vi "niFpgaFFTButterfly.vi"(0 "X in":T1, 2 "stage":u8, 5 "Y in":T1, 7 "TwiddleFactor":T1, 9 "flag":fxp<+,2,2>) -> (4 "X out":T1, 10 "Y out":T1)   [LabVIEW 2017]
uses:
  <vilib>/rvi/FXPMathLib/FxpMul/XNode/nifxpmath_Multiplier.xnode
  <vilib>/rvi/FXPMathLib/basic elements/FxpDiscreteDelay/XNode/nifxpmath_DiscreteDelay.xnode
  <vilib>/rvi/FXPMathLib/sim/FxpSim.dll
types:
  T1 = cluster{"Real":fxp<+/-,16,1>, "Imaginary":fxp<+/-,16,1>}
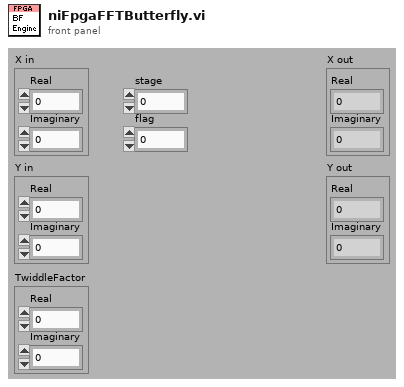
[diagram p1: front panel]
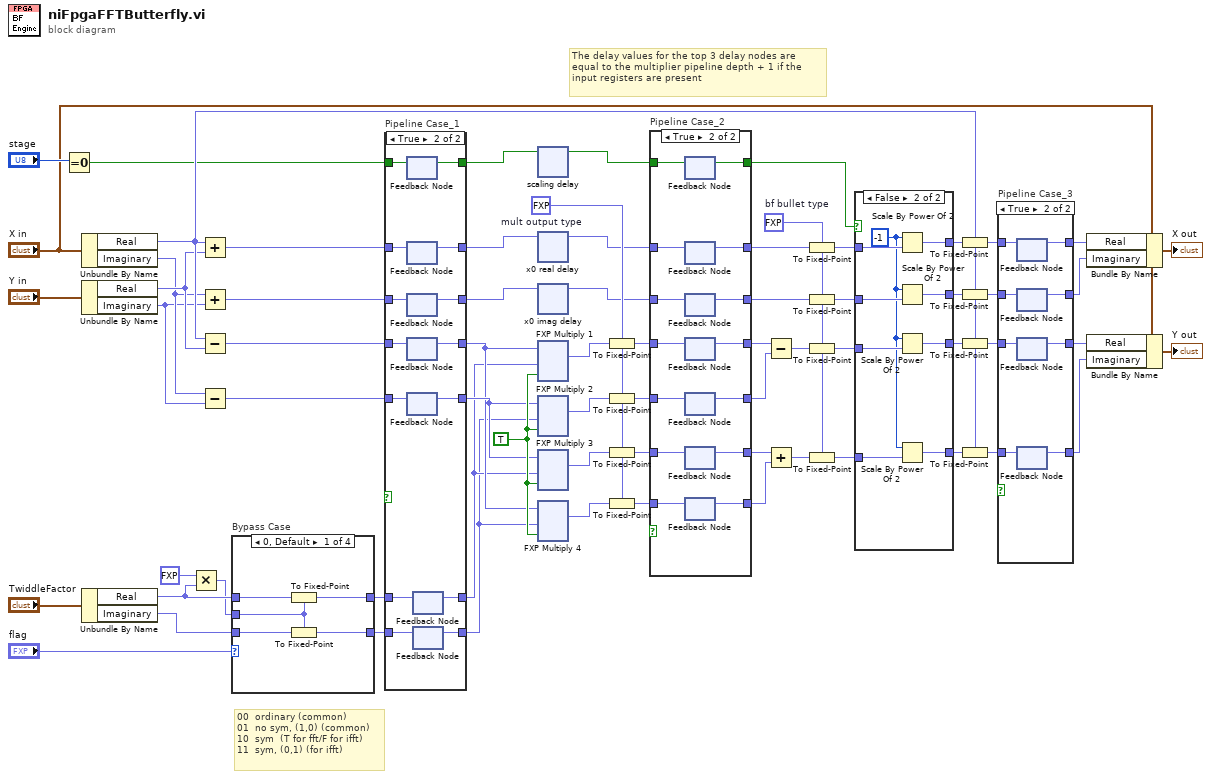
[diagram p0: block diagram]
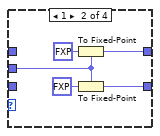
[diagram p5: hidden frame]
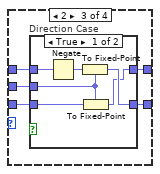
[diagram p6: hidden frame]
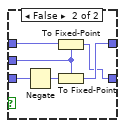
[diagram p7: hidden frame]
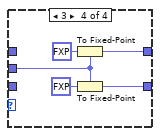
[diagram p8: hidden frame]
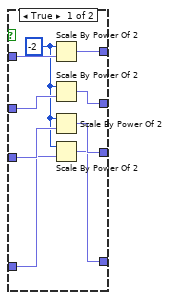
[diagram p9: hidden frame]
diagram:
  w39 = fxp<+/-,18,2> 0.0  # mult output type
  w54 = fxp<+/-,22,4> 0.0  # bf bullet type
  w38 = TRUE ("input valid")
  # "The delay values for the top 3 delay nodes are equal to the multiplier pipeline depth + 1 if the input registers are present"
  # "00  ordinary (common)\n01  no sym, (1,0) (common)\n10  sym  (T for fft/F for ifft)\n11  sym, (0,1) (for ifft)"
  n1 = Equal To 0?(x="stage") -> (x = 0?=w12:bool)
  n2 = Unbundle By Name("X in") -> ("Real"=w48:fxp<+/-,16,1>, "Imaginary"=w46:fxp<+/-,16,1>)
  n3 = Unbundle By Name("Y in") -> ("Real"=w47:fxp<+/-,16,1>, "Imaginary"=w45:fxp<+/-,16,1>)
  n4 = Unbundle By Name("TwiddleFactor") -> ("Real"=w50:fxp<+/-,16,1>, "Imaginary"=w52:fxp<+/-,16,1>)
  n5 = Multiply(x=fxp<+/-,2,2> 0.0, y=w50) -> (x*y=w49:fxp<+/-,17,2>)
  n6 = Add(x=w48, y=w47) -> (x+y=w10:fxp<+/-,17,2>)
  n7 = Add(x=w46, y=w45) -> (x+y=w9:fxp<+/-,17,2>)
  n8 = Subtract(x=w48, y=w47) -> (x-y=w29:fxp<+/-,17,2>)
  n9 = Subtract(x=w46, y=w45) -> (x-y=w30:fxp<+/-,17,2>)
  n10 = case "Bypass Case" shown="0, Default" "flag" {
    tunnel: w50 -> [w73 _ w83 _]
    tunnel: [w72 w77 w79 w99] -> w31
    tunnel: w52 -> [w71 _ w80 _]
    tunnel: [w70 w75 w82 w97] -> w32
    tunnel: w49 -> [w69 w74 w81 w96]
    frame 0, Default {
      n11 = To Fixed-Point(fixed-point type=w69, number=w73) -> (fixed-point=w72:fxp<+/-,17,2>)
      n12 = To Fixed-Point(fixed-point type=w69, number=w71) -> (fixed-point=w70:fxp<+/-,17,2>)
    }
    frame 1 {
      n13 = To Fixed-Point(fixed-point type=w74, number=fxp<+,1,1> 1.0 ("fixed-point type")) -> (fixed-point=w77:fxp<+/-,17,2>)
      n14 = To Fixed-Point(fixed-point type=w74, number=fxp<+,1,1> 0.0 ("fixed-point type")) -> (fixed-point=w75:fxp<+/-,17,2>)
    }
    frame 2 {
      n15 = case "Direction Case" shown="True" {
        selector: _ -> [_ _]
        tunnel: w83 -> [w88 w92]
        tunnel: [w87 w90] -> w82
        tunnel: w81 -> [w86 w94]
        tunnel: w80 -> [w85 w93]
        tunnel: [w84 w91] -> w79
        frame True {
          n16 = Negate(x=w88) -> (-x=w89:fxp<+/-,17,2>)
          n17 = To Fixed-Point(fixed-point type=w86, number=w89) -> (fixed-point=w87:fxp<+/-,17,2>)
          n18 = To Fixed-Point(fixed-point type=w86, number=w85) -> (fixed-point=w84:fxp<+/-,17,2>)
        }
        frame False {
          n19 = Negate(x=w93) -> (-x=w95:fxp<+/-,17,2>)
          n20 = To Fixed-Point(fixed-point type=w94, number=w92) -> (fixed-point=w90:fxp<+/-,17,2>)
          n21 = To Fixed-Point(fixed-point type=w94, number=w95) -> (fixed-point=w91:fxp<+/-,17,2>)
        }
      }
    }
    frame 3 {
      n22 = To Fixed-Point(fixed-point type=w96, number=fxp<+,1,1> 0.0 ("fixed-point type")) -> (fixed-point=w99:fxp<+/-,17,2>)
      n23 = To Fixed-Point(fixed-point type=w96, number=fxp<+,1,1> 1.0 ("fixed-point type")) -> (fixed-point=w97:fxp<+/-,17,2>)
    }
  }
  n24 = case "Pipeline Case_1" shown="True" {
    selector: _ -> [_ _]
    tunnel: [w106 w121] -> w36
    tunnel: [w107 w120] -> w35
    tunnel: [w105 w119] -> w34
    tunnel: [w104 w118] -> w33
    tunnel: w32 -> [w104 w117]
    tunnel: w31 -> [w105 w116]
    tunnel: w30 -> [w106 w115]
    tunnel: w29 -> [w107 w114]
    tunnel: w12 -> [w103 w113]
    tunnel: [w103 w112] -> w11
    tunnel: w10 -> [w102 w111]
    tunnel: w9 -> [w101 w110]
    tunnel: [w102 w109] -> w8
    tunnel: [w101 w108] -> w7
    frame False {
    }
    frame True {
      n25 = feedback-in #1(w113) -> ()
      n26 = feedback #1() -> (w112:bool)  [unwired: 1 in]
      n27 = feedback-in #2(w111) -> ()
      n28 = feedback #2() -> (w109:fxp<+/-,17,2>)  [unwired: 1 in]
      n29 = feedback-in #3(w110) -> ()
      n30 = feedback #3() -> (w108:fxp<+/-,17,2>)  [unwired: 1 in]
      n31 = feedback-in #4(w114) -> ()
      n32 = feedback #4() -> (w120:fxp<+/-,17,2>)  [unwired: 1 in]
      n33 = feedback-in #5(w115) -> ()
      n34 = feedback #5() -> (w121:fxp<+/-,17,2>)  [unwired: 1 in]
      n35 = feedback-in #6(w116) -> ()
      n36 = feedback #6() -> (w119:fxp<+/-,17,2>)  [unwired: 1 in]
      n37 = feedback-in #7(w117) -> ()
      n38 = feedback #7() -> (w118:fxp<+/-,17,2>)  [unwired: 1 in]
    }
  }
  n39 = xnode "scaling delay"("D"=w11) -> ("Q"=w5:bool)
  n40 = xnode "x0 real delay"("D"=w8) -> ("Q"=w3:fxp<+/-,17,2>)
  n41 = xnode "x0 imag delay"("D"=w7) -> ("Q"=w1:fxp<+/-,17,2>)
  n42 = xnode "FXP Multiply 1"("x"=w35, "y"=w34, "input valid"=w38) -> ("x*y"=w37:fxp<+/-,34,4>)  [unwired: 1 in, 2 out]
  n43 = xnode "FXP Multiply 2"("x"=w36, "y"=w33, "input valid"=w38) -> ("x*y"=w44:fxp<+/-,34,4>)  [unwired: 1 in, 2 out]
  n44 = xnode "FXP Multiply 3"("x"=w36, "y"=w34, "input valid"=w38) -> ("x*y"=w43:fxp<+/-,34,4>)  [unwired: 1 in, 2 out]
  n45 = xnode "FXP Multiply 4"("x"=w35, "y"=w33, "input valid"=w38) -> ("x*y"=w42:fxp<+/-,34,4>)  [unwired: 1 in, 2 out]
  n46 = To Fixed-Point(fixed-point type=w39, number=w37) -> (fixed-point=w28:fxp<+/-,18,2>)
  n47 = To Fixed-Point(fixed-point type=w39, number=w44) -> (fixed-point=w25:fxp<+/-,18,2>)
  n48 = To Fixed-Point(fixed-point type=w39, number=w43) -> (fixed-point=w24:fxp<+/-,18,2>)
  n49 = To Fixed-Point(fixed-point type=w39, number=w42) -> (fixed-point=w21:fxp<+/-,18,2>)
  n50 = case "Pipeline Case_2" shown="True" {
    selector: _ -> [_ _]
    tunnel: w28 -> [w128 w142]
    tunnel: [w128 w141] -> w27
    tunnel: [w127 w140] -> w26
    tunnel: w25 -> [w127 w139]
    tunnel: w24 -> [w126 w138]
    tunnel: [w126 w137] -> w23
    tunnel: [w125 w136] -> w22
    tunnel: w21 -> [w125 w135]
    tunnel: [w122 w133] -> w6
    tunnel: w5 -> [w122 w134]
    tunnel: [w123 w131] -> w4
    tunnel: w3 -> [w123 w132]
    tunnel: [w124 w129] -> w2
    tunnel: w1 -> [w124 w130]
    frame False {
    }
    frame True {
      n51 = feedback-in #8(w134) -> ()
      n52 = feedback #8() -> (w133:bool)  [unwired: 1 in]
      n53 = feedback-in #9(w132) -> ()
      n54 = feedback #9() -> (w131:fxp<+/-,17,2>)  [unwired: 1 in]
      n55 = feedback-in #10(w130) -> ()
      n56 = feedback #10() -> (w129:fxp<+/-,17,2>)  [unwired: 1 in]
      n57 = feedback-in #11(w142) -> ()
      n58 = feedback #11() -> (w141:fxp<+/-,18,2>)  [unwired: 1 in]
      n59 = feedback-in #12(w139) -> ()
      n60 = feedback #12() -> (w140:fxp<+/-,18,2>)  [unwired: 1 in]
      n61 = feedback-in #13(w138) -> ()
      n62 = feedback #13() -> (w137:fxp<+/-,18,2>)  [unwired: 1 in]
      n63 = feedback-in #14(w135) -> ()
      n64 = feedback #14() -> (w136:fxp<+/-,18,2>)  [unwired: 1 in]
    }
  }
  n65 = Subtract(x=w27, y=w26) -> (x-y=w41:fxp<+/-,19,3>)
  n66 = Add(x=w23, y=w22) -> (x+y=w40:fxp<+/-,19,3>)
  n67 = To Fixed-Point(fixed-point type=w54, number=w4) -> (fixed-point=w55:fxp<+/-,22,4>)
  n68 = To Fixed-Point(fixed-point type=w54, number=w2) -> (fixed-point=w56:fxp<+/-,22,4>)
  n69 = To Fixed-Point(fixed-point type=w54, number=w41) -> (fixed-point=w57:fxp<+/-,22,4>)
  n70 = To Fixed-Point(fixed-point type=w54, number=w40) -> (fixed-point=w58:fxp<+/-,22,4>)
  n71 = case shown="False" w6 {
    tunnel: w55 -> [w151 w160]
    tunnel: w56 -> [w150 w159]
    tunnel: w57 -> [w149 w158]
    tunnel: w58 -> [w148 w157]
    tunnel: [w147 w156] -> w64
    tunnel: [w146 w155] -> w63
    tunnel: [w145 w154] -> w62
    tunnel: [w144 w153] -> w61
    frame True {
      w143 = i8 -2 ("n")
      n72 = Scale By Power Of 2(n=w143, x=w151) -> (x*2^n=w144:fxp<+/-,22,4>)
      n73 = Scale By Power Of 2(n=w143, x=w150) -> (x*2^n=w145:fxp<+/-,22,4>)
      n74 = Scale By Power Of 2(n=w143, x=w149) -> (x*2^n=w147:fxp<+/-,22,4>)
      n75 = Scale By Power Of 2(n=w143, x=w148) -> (x*2^n=w146:fxp<+/-,22,4>)
    }
    frame False {
      w152 = i8 -1 ("n")
      n76 = Scale By Power Of 2(n=w152, x=w160) -> (x*2^n=w153:fxp<+/-,22,4>)
      n77 = Scale By Power Of 2(n=w152, x=w159) -> (x*2^n=w154:fxp<+/-,22,4>)
      n78 = Scale By Power Of 2(n=w152, x=w158) -> (x*2^n=w156:fxp<+/-,22,4>)
      n79 = Scale By Power Of 2(n=w152, x=w157) -> (x*2^n=w155:fxp<+/-,22,4>)
    }
  }
  n80 = To Fixed-Point(fixed-point type=w48, number=w61) -> (fixed-point=w20:fxp<+/-,16,1>)
  n81 = To Fixed-Point(fixed-point type=w48, number=w62) -> (fixed-point=w17:fxp<+/-,16,1>)
  n82 = To Fixed-Point(fixed-point type=w48, number=w64) -> (fixed-point=w16:fxp<+/-,16,1>)
  n83 = To Fixed-Point(fixed-point type=w48, number=w63) -> (fixed-point=w14:fxp<+/-,16,1>)
  n84 = case "Pipeline Case_3" shown="True" {
    selector: _ -> [_ _]
    tunnel: w20 -> [w164 w172]
    tunnel: [w164 w171] -> w19
    tunnel: [w163 w170] -> w18
    tunnel: w17 -> [w163 w169]
    tunnel: w16 -> [w162 w168]
    tunnel: [w162 w167] -> w15
    tunnel: w14 -> [w161 w166]
    tunnel: [w161 w165] -> w13
    frame False {
    }
    frame True {
      n85 = feedback-in #15(w172) -> ()
      n86 = feedback #15() -> (w171:fxp<+/-,16,1>)  [unwired: 1 in]
      n87 = feedback-in #16(w169) -> ()
      n88 = feedback #16() -> (w170:fxp<+/-,16,1>)  [unwired: 1 in]
      n89 = feedback-in #17(w168) -> ()
      n90 = feedback #17() -> (w167:fxp<+/-,16,1>)  [unwired: 1 in]
      n91 = feedback-in #18(w166) -> ()
      n92 = feedback #18() -> (w165:fxp<+/-,16,1>)  [unwired: 1 in]
    }
  }
  n93 = Bundle By Name(cluster="X in", "Real"=w19, "Imaginary"=w18) -> (→"X out":T1)
  n94 = Bundle By Name(cluster="X in", "Real"=w15, "Imaginary"=w13) -> (→"Y out":T1)
